vi "CRC16.vi"(0 "待计算数组":u8[](array[numeric]) format="%x", 1 "CRC码":u16 format="%x") -> (2 "CRC_H":u8 format="%x", 3 "CRC_L":u8 format="%x")   [LabVIEW 2009]
panel:
  in  "CRC_表":u16[](array[numeric]) format="%x"
  out "ucTemp":u8 format="%x"
  # "0x8108,0x9129,0xA14A,0xB16B,0xC18C,0xD1AD,0xE1CE,0xF1EF"
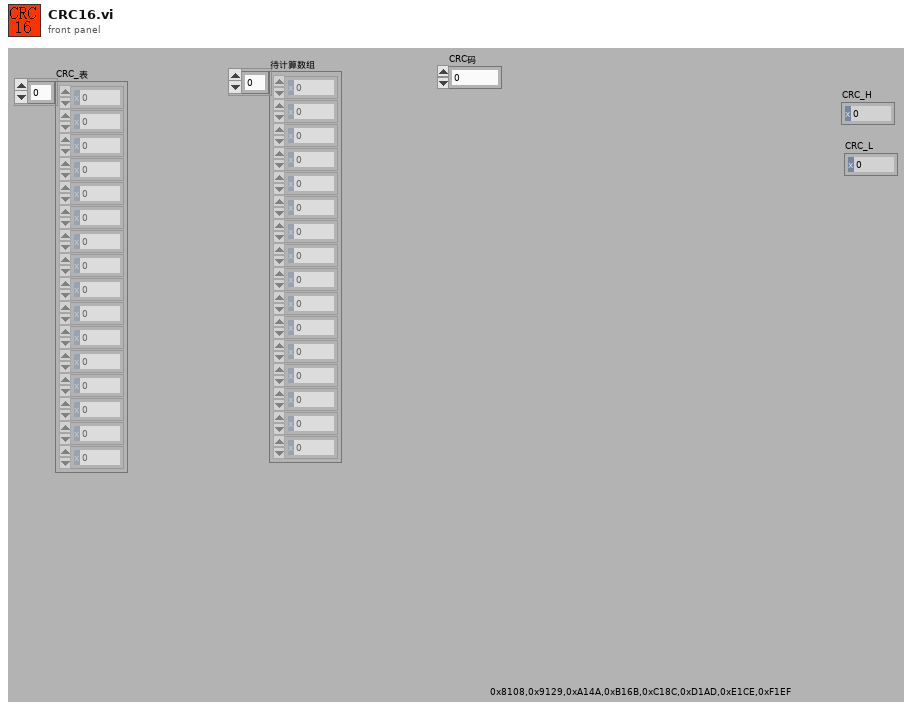
[diagram p1: front panel]
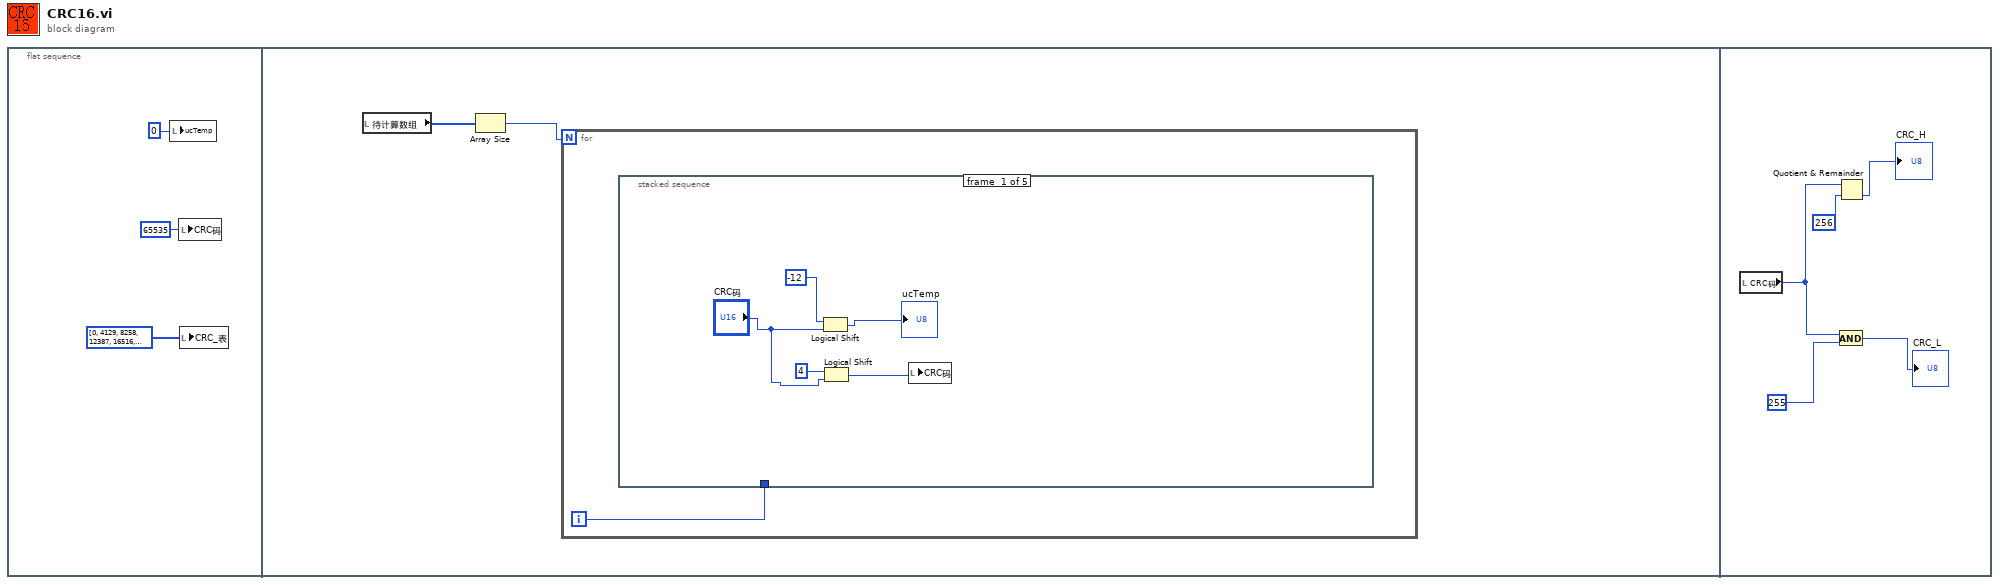
[diagram p0: block diagram]
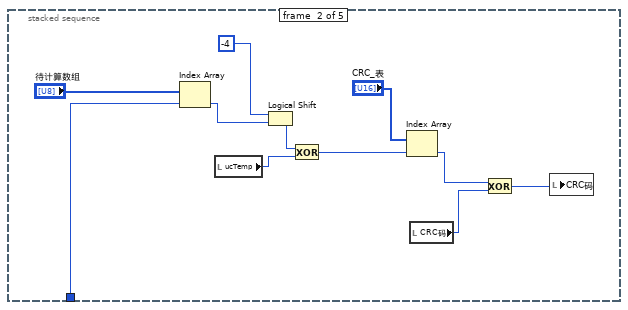
[diagram p2: hidden frame]
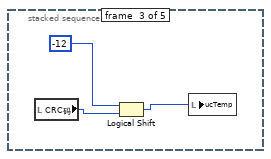
[diagram p3: hidden frame]
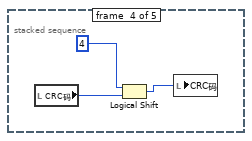
[diagram p4: hidden frame]
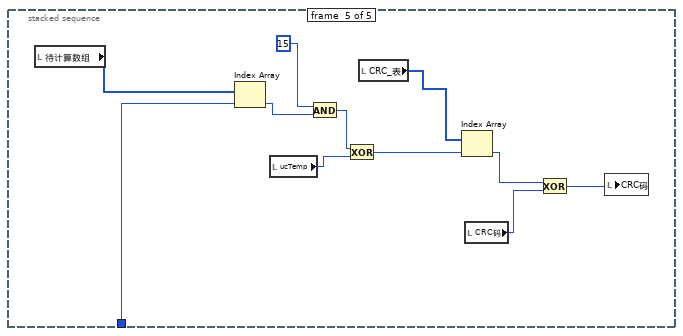
[diagram p5: hidden frame]
diagram:
  n1 = flat-sequence {
    frame #0 {
      n2 = local write "ucTemp"(u8 0 ("ucTemp")) -> ()
      n3 = local write "CRC码"(u16 65535 ("uwCRC")) -> ()
      n4 = local write "CRC_表"(u16[] [0, 4129, 8258, 12387, 16516, 20645, 24774, 28903, 33032, 37161, 41290, 45419, 49548, 53677, 57806, 61935] ("CRC_TABLE")) -> ()
    }
    frame #1 {
      n5 = local read "待计算数组"() -> (w4:u8[])
      n6 = Array Size(array=w4) -> (size(s)=w5:i32)
      n7 = for {
        N: w5 -> [_]
        i -> [w6]
        n8 = stacked-sequence {
          tunnel: w6 -> [_ w21 _ _ w34]
          frame #0 {
            n9 = Logical Shift(y=i16 -12, x="CRC码") -> (x << y=→"ucTemp":u16)
            n10 = Logical Shift(y=i16 4, x="CRC码") -> (x << y=w11:u16)
            n11 = local write "CRC码"(w11) -> ()
          }
          frame #1 {
            n12 = Index Array(array="待计算数组", index=w21) -> (element=w12:u8)
            n13 = local read "ucTemp"() -> (w15:u8)
            n14 = Logical Shift(y=i16 -4, x=w12) -> (x << y=w14:u8)
            n15 = Exclusive Or(1:w15, 2:w14) -> (0:w17:u8)
            n16 = Index Array(array="CRC_表", index=w17) -> (element=w19:u16)
            n17 = local read "CRC码"() -> (w18:u16)
            n18 = Exclusive Or(1:w18, 2:w19) -> (0:w20:u16)
            n19 = local write "CRC码"(w20) -> ()
          }
          frame #2 {
            n20 = local read "CRC码"() -> (w24:u16)
            n21 = Logical Shift(y=i16 -12, x=w24) -> (x << y=w23:u16)
            n22 = local write "ucTemp"(w23) -> ()
          }
          frame #3 {
            n23 = local read "CRC码"() -> (w27:u16)
            n24 = Logical Shift(y=i8 4 ("x << y"), x=w27) -> (x << y=w28:u16)
            n25 = local write "CRC码"(w28) -> ()
          }
          frame #4 {
            n26 = local read "待计算数组"() -> (w29:u8[])
            n27 = Index Array(array=w29, index=w34) -> (element=w32:u8)
            n28 = local read "ucTemp"() -> (w35:u8)
            n29 = And(x=u8 15 ("y"), y=w32) -> (x .and. y?=w31:u8)
            n30 = Exclusive Or(1:w35, 2:w31) -> (0:w36:u8)
            n31 = local read "CRC_表"() -> (w30:u16[])
            n32 = Index Array(array=w30, index=w36) -> (element=w38:u16)
            n33 = local read "CRC码"() -> (w37:u16)
            n34 = Exclusive Or(1:w37, 2:w38) -> (0:w39:u16)
            n35 = local write "CRC码"(w39) -> ()
          }
        }
      }
    }
    frame #2 {
      n36 = local read "CRC码"() -> (w42:u16)
      n37 = And(x=w42, y=u16 255) -> (x .and. y?=→"CRC_L":u16)
      n38 = Quotient & Remainder(x=w42, y=u16 256) -> (floor(x/y)=→"CRC_H":u16)  [unwired: 1 out]
    }
  }
